vi "AverageOneCoord (SubVI).vi"(0 "Array":dbl[](array[numeric])) -> (4 "Top averages":dbl[][](array[numeric]), 6 "Bottom averages":dbl[][](array[numeric]), 8 "Top SD":dbl[][](array[numeric]), 10 "Bottom SD":dbl[][](array[numeric]))   [LabVIEW 2016]
uses:
  <vilib>/Analysis/NI_AALBase.lvlib
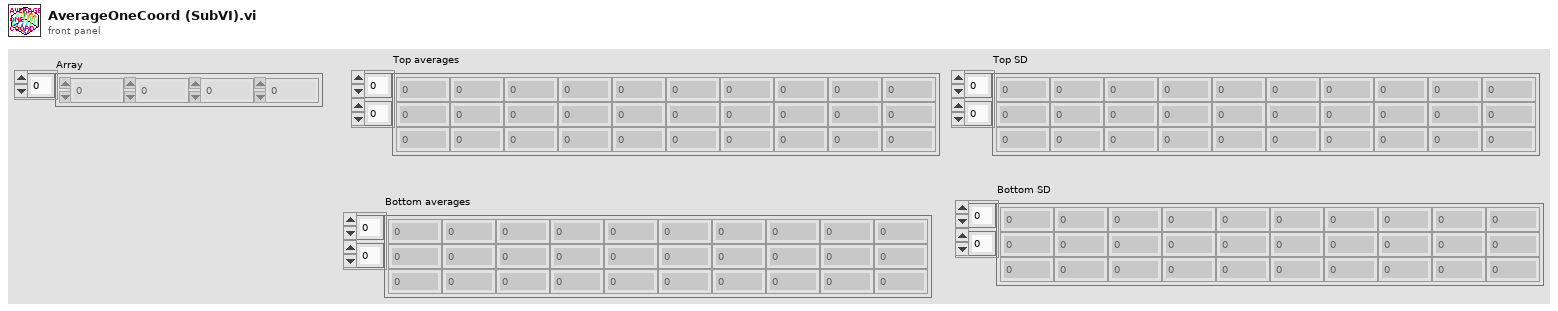
[diagram p1: front panel]
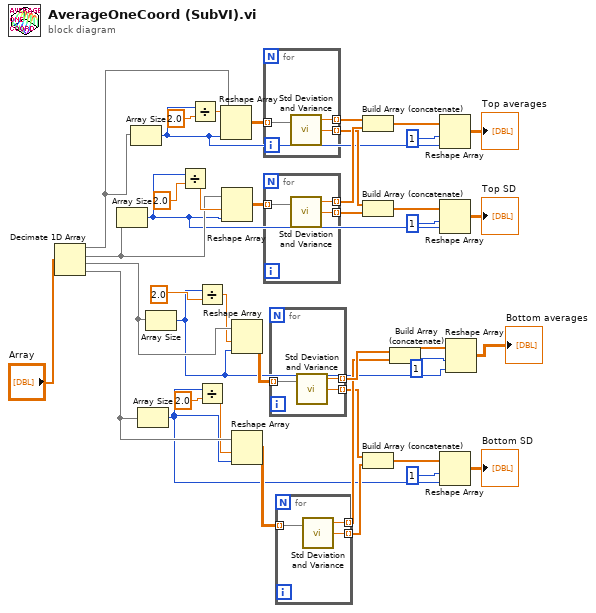
[diagram p0: block diagram]
diagram:
  n1 = Decimate 1D Array("Array") -> (w16:dbl[], w9:dbl[], w8:dbl[], w6:dbl[])
  n2 = Array Size(array=w9) -> (size(s)=w3:i32)
  n3 = Array Size(array=w16) -> (size(s)=w4:i32)
  n4 = Array Size(array=w6) -> (size(s)=w1:i32)
  n5 = Array Size(array=w8) -> (size(s)=w2:i32)
  n6 = Divide(x=w3, y=2.0) -> (x/y=w10:dbl)
  n7 = Divide(x=w4, y=2.0) -> (x/y=w14:dbl)
  n8 = Divide(x=w2, y=2.0) -> (x/y=w7:dbl)
  n9 = Divide(x=w1, y=2.0) -> (x/y=w5:dbl)
  n10 = Reshape Array(w16, w14, w4) -> (w40:dbl[][])
  n11 = Reshape Array(w9, w10, w3) -> (w39:dbl[][])
  n12 = Reshape Array(w8, w7, w2) -> (w38:dbl[][])
  n13 = Reshape Array(w6, w5, w1) -> (w37:dbl[][])
  n14 = for {
    tunnel: w40 -> [w44] mode=indexing
    tunnel: [w43] -> w36 mode=indexing
    tunnel: [w42] -> w22 mode=indexing
    n15 = call <vilib>:"Std Deviation and Variance.vi"("X"=w44) -> ("mean"=w43:dbl, "standard deviation"=w42:dbl)  [unwired: 1 in, 1 out]
  }
  n16 = for {
    tunnel: w39 -> [w47] mode=indexing
    tunnel: [w46] -> w35 mode=indexing
    tunnel: [w45] -> w21 mode=indexing
    n17 = call <vilib>:"Std Deviation and Variance.vi"("X"=w47) -> ("mean"=w46:dbl, "standard deviation"=w45:dbl)  [unwired: 1 in, 1 out]
  }
  n18 = for {
    tunnel: w38 -> [w50] mode=indexing
    tunnel: [w49] -> w20 mode=indexing
    tunnel: [w48] -> w18 mode=indexing
    n19 = call <vilib>:"Std Deviation and Variance.vi"("X"=w50) -> ("mean"=w49:dbl, "standard deviation"=w48:dbl)  [unwired: 1 in, 1 out]
  }
  n20 = for {
    tunnel: w37 -> [w53] mode=indexing
    tunnel: [w52] -> w19 mode=indexing
    tunnel: [w51] -> w17 mode=indexing
    n21 = call <vilib>:"Std Deviation and Variance.vi"("X"=w53) -> ("mean"=w52:dbl, "standard deviation"=w51:dbl)  [unwired: 1 in, 1 out]
  }
  n22 = Build Array (concatenate)(w36, w35) -> (w34:dbl[])
  n23 = Build Array (concatenate)(w22, w21) -> (w31:dbl[])
  n24 = Build Array (concatenate)(w18, w17) -> (w25:dbl[])
  n25 = Build Array (concatenate)(w20, w19) -> (w28:dbl[])
  n26 = Reshape Array(w34, 1 ("dimension size"), w4) -> (→"Top averages":dbl[][])
  n27 = Reshape Array(w31, 1 ("dimension size"), w3) -> (→"Top SD":dbl[][])
  n28 = Reshape Array(w25, 1 ("dimension size"), w1) -> (→"Bottom SD":dbl[][])
  n29 = Reshape Array(w28, 1 ("dimension size"), w2) -> (→"Bottom averages":dbl[][])
